vi "ClearDisconnectError.vi"(8 "error in (no error)":errorcluster) -> (0 "error out":errorcluster, 3 "Disconnect error?":bool)   [LabVIEW 2013]
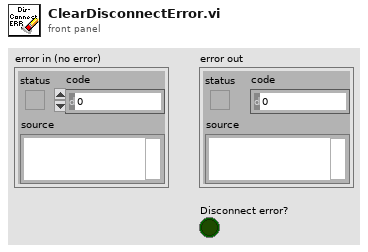
[diagram p1: front panel]
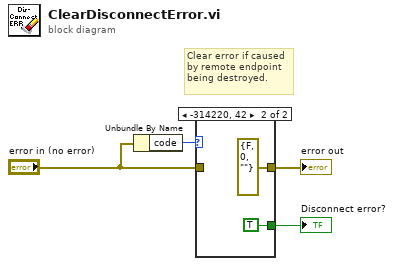
[diagram p0: block diagram]
diagram:
  # "Clear error if caused\nby remote endpoint\nbeing destroyed."
  n1 = Unbundle By Name("error in (no error)") -> ("code"=w2:i32)
  n2 = case shown="-314220, 42" w2 {
    tunnel: "error in (no error)" -> [w5 _]
    tunnel: [w5 errorcluster {"status"=FALSE, "code"=0, "source"=""} ("error out")] -> w4
    tunnel: [_ TRUE ("status")] -> w1
    frame 0, Default {
    }
    frame -314220, 42 {
    }
  }
  "error out" <- w4
  "Disconnect error?" <- w1
